vi "Jog.vi"(8 "error in (no error)":errorcluster, 9 "Jog Negative":bool, 10 "Jog Positive":bool, 11 "FHPP in":refnum<class "FHPP.lvclass">) -> (0 "error out":errorcluster, 3 "FHPP out":refnum<class "FHPP.lvclass">)   [LabVIEW 2022 SP3, in "FHPP.lvclass"]
uses:
  FHPP.lvclass
  FHPP.lvclass/FHPP.ctl
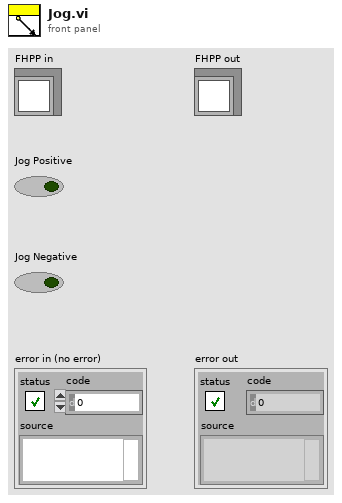
[diagram p1: front panel]
types:
  T1 = typedef "FHPP.lvclass/CPOS.ctl" = cluster{"Halt":bool, "Start":bool, "Start Homing":bool, "Jog Positive":bool, "Jog Negative":bool, "Teach Actual Value":bool, "Clear Remaining Pos":bool, "Reserved":bool}
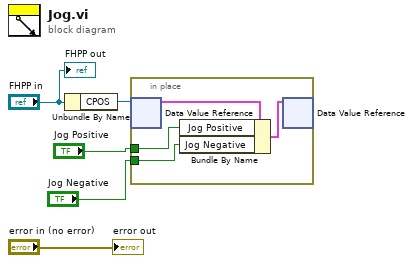
[diagram p0: block diagram]
diagram:
  n1 = Unbundle By Name("FHPP in") -> ("CPOS"=w3:refnum<data-value>)
  n2 = in-place {
    in-place-border: "Jog Positive" -> [w7]
    in-place-border: "Jog Negative" -> [w6]
    n3 = in-place-dvr #1(w3) -> (w9:T1)  [unwired: 1 out]
    n4 = Bundle By Name(cluster=w9, "Jog Positive"=w7, "Jog Negative"=w6) -> (w8:T1)
    n5 = in-place-dvr #1(w8) -> ()  [unwired: 2 out]
  }
  "error out" <- "error in (no error)"
  "FHPP out" <- "FHPP in"
